vi "Update Histogram Visibility.vi"(6 "DisplayMode":T1, 8 "error in (no error)":errorcluster, 11 "Instruments in":refnum<class "Instruments.lvclass">) -> (0 "error out":errorcluster, 3 "Instruments out":refnum<class "Instruments.lvclass">)   [LabVIEW 2023, in "Instruments.lvlib" / "Instruments.lvclass"]
doc: "Sets Waveform Display Visibility to true when display mode is Histogram"
uses:
  Library/Instruments.lvclass
  Custom Controls/Display Mode.ctl
  Library/Instruments.lvclass/Instruments.ctl
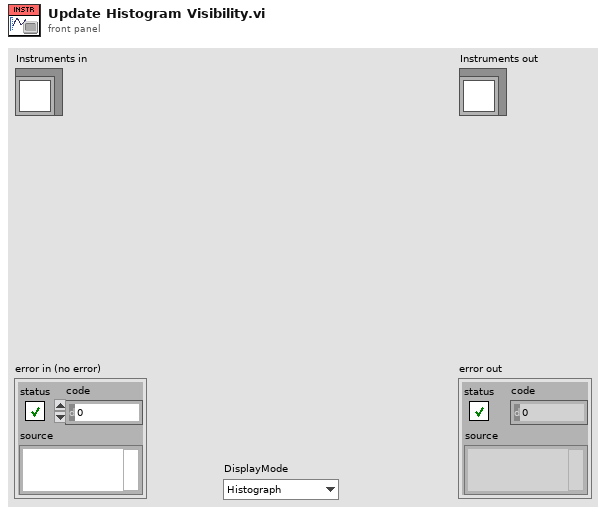
[diagram p1: front panel]
types:
  T1 = typedef "Instruments.lvlib/Instruments.lvclass/Display Mode.ctl" = enum16{"Histograph", "Table", "Snapshot"}
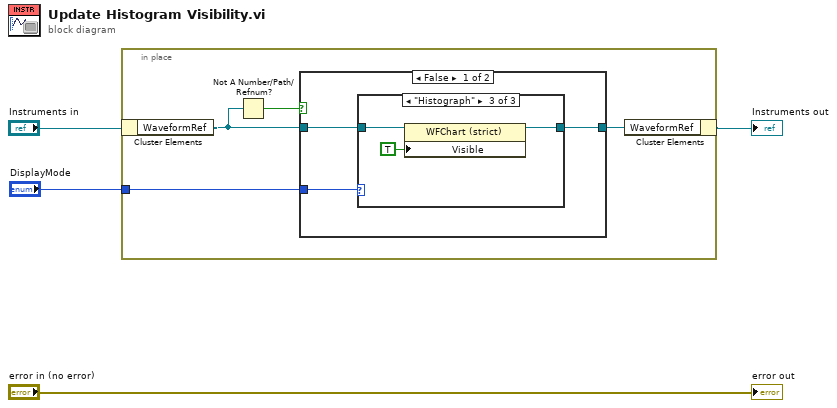
[diagram p0: block diagram]
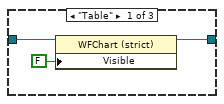
[diagram p2: hidden frame]
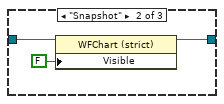
[diagram p3: hidden frame]
diagram:
  n1 = in-place {
    in-place-border: "DisplayMode" -> [w5]
    n2 = in-place-cluster #1("Instruments in") -> ("WaveformRef"=w7:refnum<vi>)
    n3 = Not A Number/Path/Refnum?(number/path/refnum=w7) -> (NaN/Path/Refnum?=w6:bool)
    n4 = case shown="False" w6 {
      tunnel: [w11 w21] -> w8
      tunnel: w7 -> [w10 w21]
      tunnel: w5 -> [w9 _]
      frame False {
        n5 = case shown="\"Histograph\"" w9 {
          tunnel: [w14 w17 w20] -> w11
          tunnel: w10 -> [w13 w16 w19]
          frame "Table" {
            n6 = property class="WFChart (strict)"(reference=w13, "Visible"=FALSE) -> (reference out=w14:refnum<vi>)  [unwired: 1 in, 1 out]
          }
          frame "Snapshot" {
            n7 = property class="WFChart (strict)"(reference=w16, "Visible"=FALSE) -> (reference out=w17:refnum<vi>)  [unwired: 1 in, 1 out]
          }
          frame "Histograph" {
            n8 = property class="WFChart (strict)"(reference=w19, "Visible"=TRUE) -> (reference out=w20:refnum<vi>)  [unwired: 1 in, 1 out]
          }
        }
      }
      frame True {
      }
    }
    n9 = in-place-cluster #1("WaveformRef"=w8) -> (→"Instruments out":refnum<class "Instruments.lvclass">)
  }
  "error out" <- "error in (no error)"
